vi "Initialize.vi"(8 "error in (no error)":errorcluster) -> (0 "error out":errorcluster)   [LabVIEW 2018, in "lvwpcap.lvlib"]
doc: "This VI initializes the packet sniffer routine."
uses:
  lvwpcap.lvlib
  lvwpcap.dll
panel:
  # "Select Help»Show Context Help and move the cursor over the VI icon to display help for this VI."
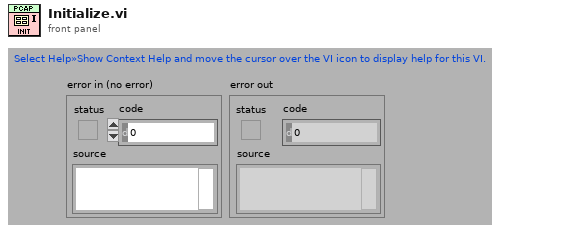
[diagram p1: front panel]
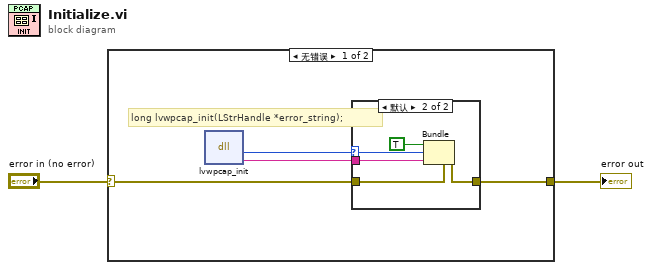
[diagram p0: block diagram]
diagram:
  n1 = case shown="无错误" "error in (no error)" {
    selector: "error in (no error)" -> [w3 w13]
    tunnel: [w4 w13] -> w2
    frame No Error {
      # "long lvwpcap_init(LStrHandle *error_string);"
      n2 = dll-call lib="PTH2:abs G论坛资料packet_sniffer_projectlvwpcap.dll" fn="lvwpcap_init"() -> (w6:i32, "error_string"=w5:string)  [unwired: 4 in, 2 out]
      n3 = case shown="默认" w6 {
        selector: w6 -> [_ w11]
        tunnel: w5 -> [_ w10]
        tunnel: w3 -> [w7 w12]
        tunnel: [w7 w8] -> w4
        frame 0 {
        }
        frame Default {
          n4 = Bundle(cluster=w12, "status"=TRUE, "code"=w11, "source"=w10) -> (w8:errorcluster)
        }
      }
    }
    frame Error {
    }
  }
  "error out" <- w2
